vi "柱塞泵KB读取.vi"(7 "是否启用通讯通知":bool, 8 "error in (no error)":errorcluster, 11 "Slave ID":T1) -> (0 "error out":errorcluster, 2 "B":sgl, 3 "K":sgl)   [LabVIEW 2016, in "质控单元V1.lvlib"]
uses:
  <vilib>/Plasmionique/MB Master/MB_Master/MB_Master.lvclass
  <vilib>/Plasmionique/MB Master/MB Master.lvlib
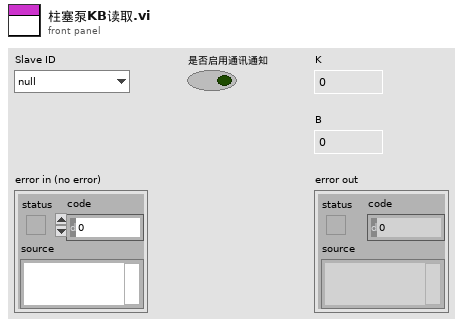
[diagram p1: front panel]
types:
  T1 = typedef "质控单元V1.lvlib/质控slave id.ctl" = enum16{"null", "氨氮", "总磷", "CODMn", "CODCr", "总氮"}
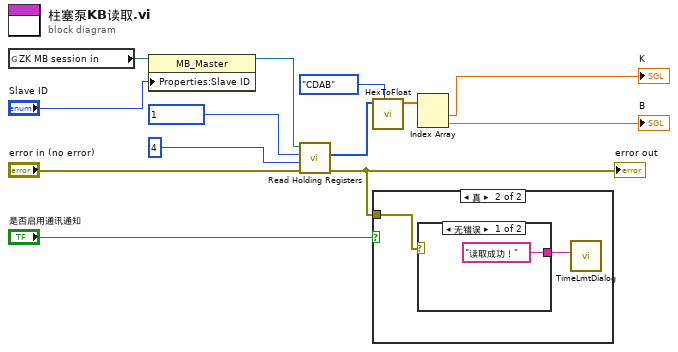
[diagram p0: block diagram]
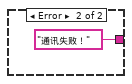
[diagram p3: hidden frame]
diagram:
  n1 = global read "ZK非断电保存全局变量.vi" "ZK MB session in"() -> (w12:refnum<class "MB_Master.lvclass">)
  n2 = property class="MB_Master"(reference=w12, "Properties:Slave ID"="Slave ID") -> (reference out=w10:refnum<class "MB_Master.lvclass">)  [unwired: 1 in, 1 out]
  n3 = call <vilib>:"Read Holding Registers.vi"("error in (no error)"="error in (no error)", "quantity"=u16 4, "starting address"=u16 1, "MB session in"=w10) -> ("error out"=w3:errorcluster, "Registers"=w7:u16[])  [unwired: 5 in, 1 out]
  "error out" <- w3
  n4 = call "HexToFloat.vi"("转换类型"=enum16{"DCBA", "CDAB"}."CDAB", "数组"=w7) -> ("FLOAT"=w6:sgl[])  [unwired: 9 in]
  n5 = case shown="真" "是否启用通讯通知" {
    tunnel: w3 -> [_ w15]
    frame False {
    }
    frame True {
      n6 = case shown="无错误" w15 {
        tunnel: ["读取成功！" "通讯失败！"] -> w14
        frame No Error {
        }
        frame Error {
        }
      }
      n7 = call "TimeLmtDialog.vi"("Infoin"=w14) -> ()  [unwired: 11 in]
    }
  }
  n8 = Index Array(array=w6) -> (element #1=→"K":sgl, element #2=→"B":sgl)  [unwired: 2 in]
